vi "IntersecPlanePts.vi"(0 "circles":i32=1, 1 "P":cluster{"x":dbl, "y":dbl, "z":dbl} {"z" format="%.2f"; "y" format="%.2f"; "x" format="%.2f"}, 2 "d":dbl format="%.2f", 3 "Sigma":dbl format="%.2f", 4 "Ring":u16(ring) items=["Circle", "Plane"], 5 "r":dbl format="%.2f") -> (6 "x matrix":dbl[][](array[numeric]) format="%.2f", 7 "y matrix":dbl[][](array[numeric]) format="%.2f", 8 "z matrix":dbl[][](array[numeric]) format="%.2f")   [LabVIEW 2022 SP3]
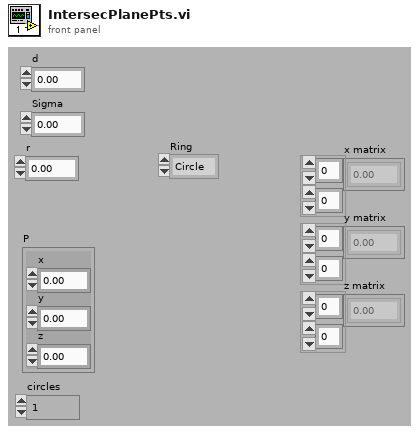
[diagram p1: front panel]
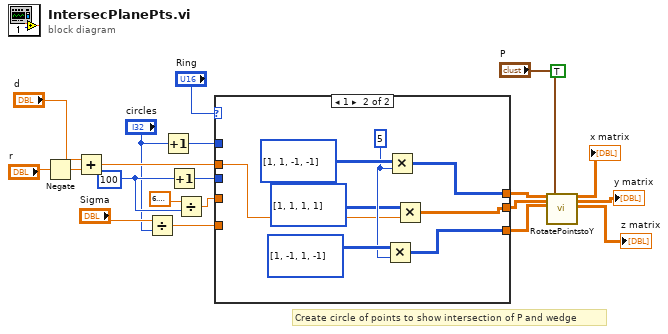
[diagram p0: block diagram]
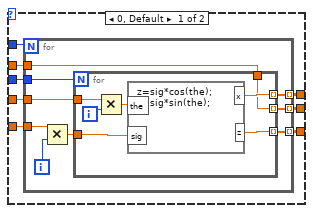
[diagram p2: hidden frame]
diagram:
  (unwired) TRUE
  w19 = 100
  # "Create circle of points to show intersection of P and wedge"
  n1 = Negate(x="r") -> (-x=w16:dbl)
  n2 = Add(x="d", y=w16) -> (x+y=w12:dbl)
  n3 = Divide(x="Sigma", y="circles") -> (x/y=w10:dbl)
  n4 = Increment(x="circles") -> (x+1=w2:i32)
  n5 = Increment(x=w19) -> (x+1=w14:i32)
  n6 = Divide(x=6.283185307179586, y=w19) -> (x/y=w13:dbl)
  n7 = case shown="1" "Ring" {
    tunnel: w14 -> [w28 _]
    tunnel: w13 -> [w27 _]
    tunnel: w12 -> [w26 w47]
    tunnel: w10 -> [w25 _]
    tunnel: [w24 w49] -> w8
    tunnel: [w23 w45] -> w7
    tunnel: [w22 w48] -> w6
    tunnel: w2 -> [w21 _]
    frame 0, Default {
      n8 = for {
        N: w21 -> [_]
        tunnel: w28 -> [w37]
        tunnel: w27 -> [w36]
        tunnel: w26 -> [w35]
        tunnel: w25 -> [w34]
        tunnel: [w33] -> w24 mode=indexing
        tunnel: [w32] -> w23 mode=indexing
        tunnel: [w31] -> w22 mode=indexing
        i -> [w29]
        n9 = Multiply(x=w34, y=w29) -> (x*y=w30:dbl)
        n10 = for {
          N: w37 -> [_]
          tunnel: [w42] -> w33 mode=indexing
          tunnel: [w41] -> w31 mode=indexing
          tunnel: w36 -> [w40]
          tunnel: w35 -> [w39]
          tunnel: [w39] -> w32 mode=indexing
          tunnel: w30 -> [w38]
          i -> [w44]
          n11 = Multiply(x=w40, y=w44) -> (x*y=w43:dbl)
          n12 = formula code="z=sig*cos(the);\nx=sig*sin(the);"("the"=w43, "sig"=w38) -> ("x"=w42:dbl, "z"=w41:dbl)
        }
      }
    }
    frame 1 {
      w50 = 5
      n13 = Multiply(x=i32[][] [[1, -1], [1, -1]], y=w50) -> (x*y=w48:i32[][])
      n14 = Multiply(x=i32[][] [[1, 1], [-1, -1]], y=w50) -> (x*y=w49:i32[][])
      n15 = Multiply(x=i32[][] [[1, 1], [1, 1]], y=w47) -> (x*y=w45:dbl[][])
    }
  }
  n16 = call "RotatePointstoY.vi"("x matrix"=w8, "y matrix"=w7, "z matrix"=w6, "P"="P") -> ("x matrix"=→"x matrix":dbl[][], "y matrix"=→"y matrix":dbl[][], "z matrix"=→"z matrix":dbl[][])  [unwired: 4 in, 9 out]
